vi "Voltperdivknob.vi"(8 "error in (no error)":errorcluster, 11 "Dial":u32(knob) scale=0.0..36.0) -> (0 "error out":errorcluster, 3 "Volt/Div.":dbl)   [LabVIEW 2014]
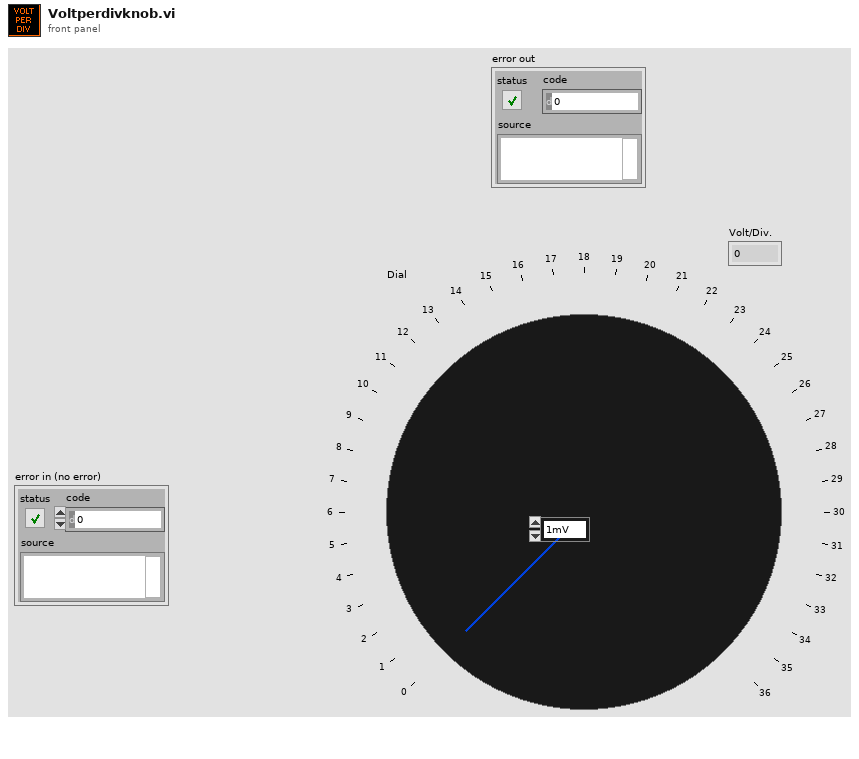
[diagram p1: front panel]
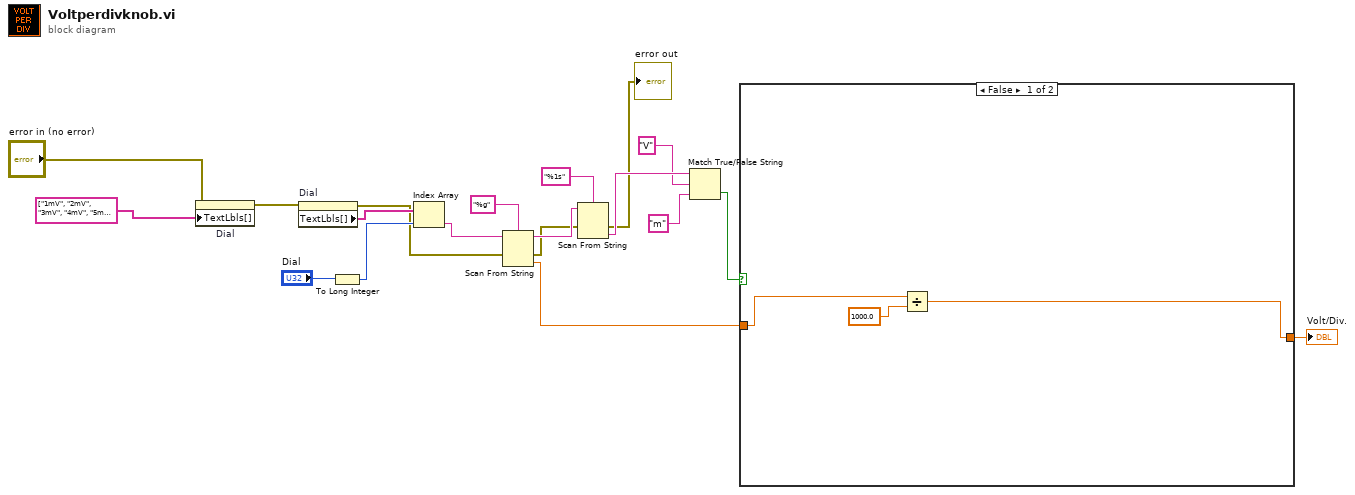
[diagram p0: block diagram]
diagram:
  n1 = property on="Dial" class="Knob (strict)"(error in="error in (no error)", "TextLbls[]"=string[] ["1mV", "2mV", "3mV", "4mV", "5mV", "6mV", "7mV", "8mV", "9mV", "10mV", "20mV", "30mV", "40mV", "50mV", "60mV", "70mV", "80mV", "90mV", "100mV", "200mV", "300mV", "400mV", "500mV", "600mV", "700mV", "800mV", "900mV", "1V", "2V", "3V", "4V", "5V", "6V", "7V", "8V", "9V", "10V"]) -> (error out=w17:errorcluster)  [unwired: 1 in, 1 out]
  n2 = property on="Dial" class="Knob (strict)"(error in=w17) -> (error out=w3:errorcluster, "TextLbls[]"=w16:string[])  [unwired: 1 in, 1 out]
  n3 = To Long Integer(number="Dial") -> (32bit integer=w4:i32)
  n4 = Index Array(array=w16, index=w4) -> (element=w14:string)
  n5 = Scan From String(format string="%g", input string=w14, error in=w3) -> (remaining string=w12:string, error out=w2:errorcluster, output 1=w7:dbl)  [unwired: 2 in, 1 out]
  n6 = Scan From String(format string="%1s", input string=w12, error in=w2) -> (error out=→"error out":errorcluster, output 1=w11:string)  [unwired: 2 in, 2 out]
  n7 = Match True/False String(2:"m" ("false string"), 3:"V" ("true string"), 4:w11) -> (0:w8:bool)  [unwired: 1 out]
  n8 = case shown="False" w8 {
    tunnel: w7 -> [w22 w23]
    tunnel: [w20 w23] -> w6
    frame False {
      n9 = Divide(x=w22, y=1000.0) -> (x/y=w20:dbl)
    }
    frame True {
    }
  }
  "Volt/Div." <- w6
